vi "Pressure Diff.vi"() -> ()   [LabVIEW 2013]
panel:
  in  "Record Data?":bool=TRUE
  out "Waveform Chart 2":dynamicdata(graph)
  out "Power":dbl
  in  "Vdot":dbl
  out "dP (Pa)":dbl
  in  "P2":dbl
  in  "P1":dbl
  out "Waveform Chart":dynamicdata(graph)
  in  "stop (F)":bool
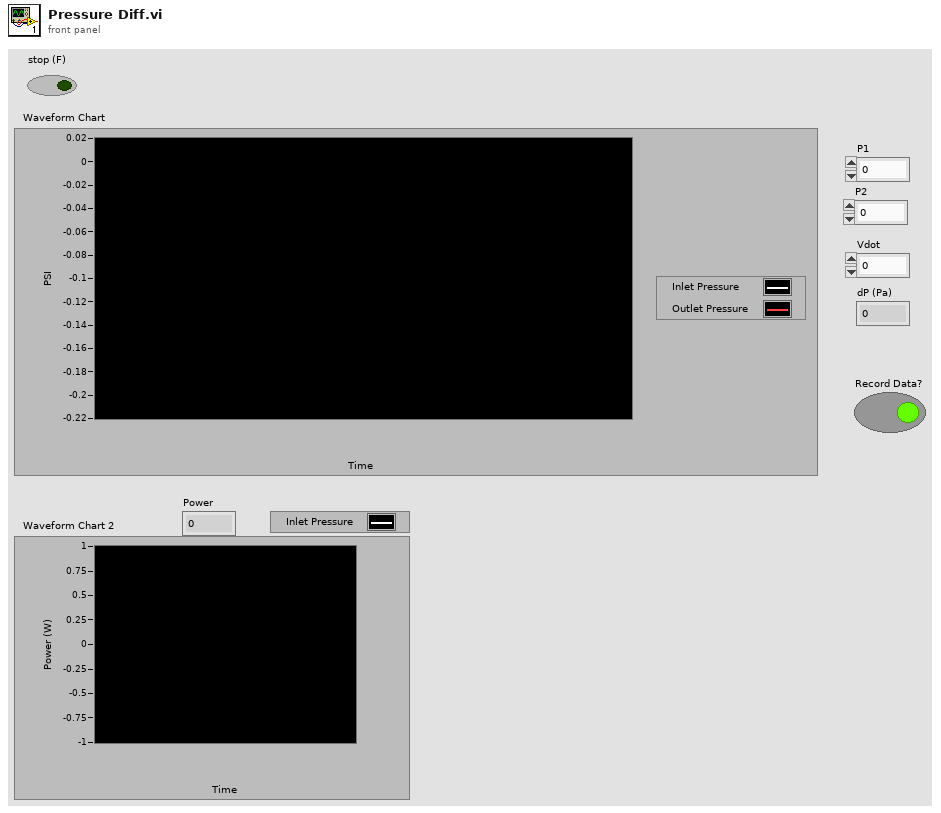
[diagram p1: front panel]
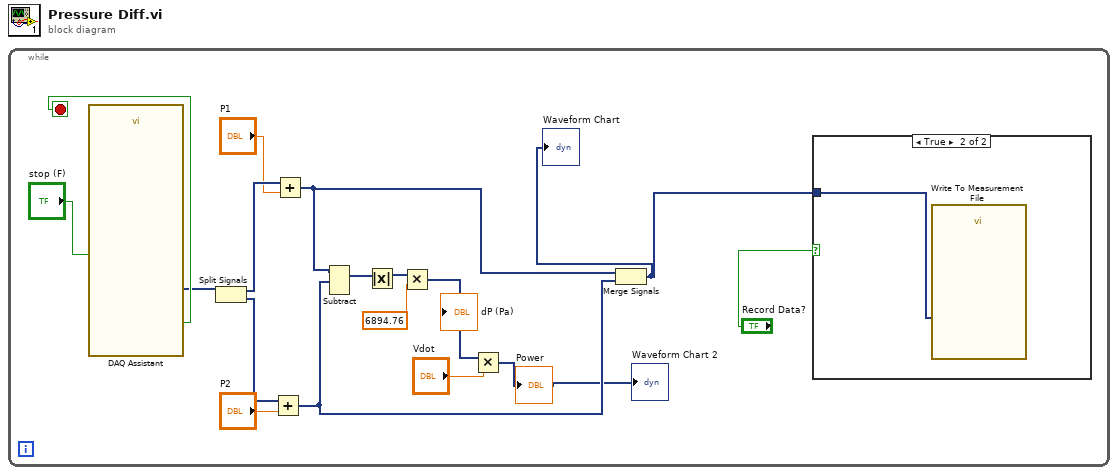
[diagram p0: block diagram]
diagram:
  n1 = while {
    stop <- w16 stop-if-true
    n2 = call "DAQ Assistant"("stop (F)"="stop (F)") -> ("data"=w15:dynamicdata, "stopped"=w16:bool)  [unwired: 15 in, 2 out]
    n3 = Split Signals(w15) -> (w14:dynamicdata, w13:dynamicdata)  [unwired: 2 in]
    n4 = Add(x=w13, y="P2") -> (x+y=w9:dynamicdata)
    n5 = Add(x=w14, y="P1") -> (x+y=w10:dynamicdata)
    n6 = Subtract(1:w9, 2:w10) -> (0:w8:dynamicdata)  [unwired: 1 in, 1 out]
    n7 = Absolute Value(x=w8) -> (abs(x)=w7:dynamicdata)
    n8 = Multiply(x=w7, y=6894.76) -> (x*y=w5:dynamicdata)
    "dP (Pa)" <- w5
    n9 = Multiply(x=w5, y="Vdot") -> (x*y=→"Power" →"Waveform Chart 2":dynamicdata)
    n10 = Merge Signals(w10, w9) -> (w1:dynamicdata)
    "Waveform Chart" <- w1
    n11 = case shown="True" "Record Data?" {
      tunnel: w1 -> [_ w18]
      frame False {
      }
      frame True {
        n12 = call "Write To Measurement File"("Signals"=w18) -> ()  [unwired: 16 in, 3 out]
      }
    }
  }
